vi "Send.vi"(10 "Error":errorcluster) -> (3 "Override Error Msg out":refnum<class "Override Error Msg.lvclass">)   [LabVIEW 2021, in "Override Error.lvlib" / "Override Error Msg.lvclass"]
uses:
  Override Error Msg.lvclass
  Override Error Msg.lvclass/Override Error Msg.ctl
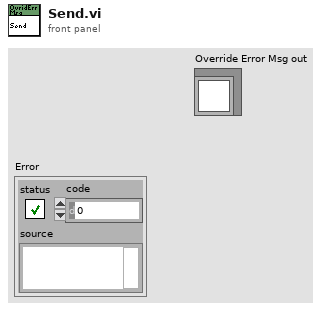
[diagram p1: front panel]
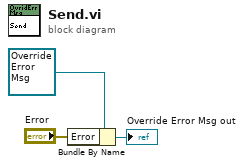
[diagram p0: block diagram]
diagram:
  n1 = Bundle By Name(cluster=refnum<class "Override Error Msg.lvclass"> refnum ("Override Error Msg out"), "Error"="Error") -> (→"Override Error Msg out":refnum<class "Override Error Msg.lvclass">)
